vi "save_config.vi"() -> ()   [LabVIEW 2013]
uses:
  <vilib>/Analysis/Matrix/Datatypes/RealMatrix.ctl
  <vilib>/Analysis/Matrix/NI_Matrix.lvlib
panel:
  in  "Version":string="f"
  in  "Camera Serial":string="f"
  in  "Camera Model":string="f"
  in  "SOFT_VERSION":string="V2"
  in  "config Name":string="test2"
  in  "Config Directory":path=path "D:/CONFIGS_TIME_LAPSE"
  in  "USED_FILTERS":u8[](array[numeric])
  in  "USED_LEDS":bool[][](array[boolean])=[[FALSE, FALSE], [TRUE, TRUE]]
  in  "Nstart":u32=30 step=1
  in  "Non":u32=150 step=1
  in  "Noff":u32 step=1
  in  "BETWEEN_PAT":u32
  in  "NPAT":u32
  in  "BETWEEN_SCAN":u32
  in  "NSCAN":u32
  in  "XYPOS":T1=[[1.0, 1.0]]
  in  "STAGE_PORT":refnum<visa-resource-name>="COM1"
  in  "STAGE_SPEED":dbl
  in  "ROMODE":u32
  in  "BIN":u16
  in  "EXPT":dbl
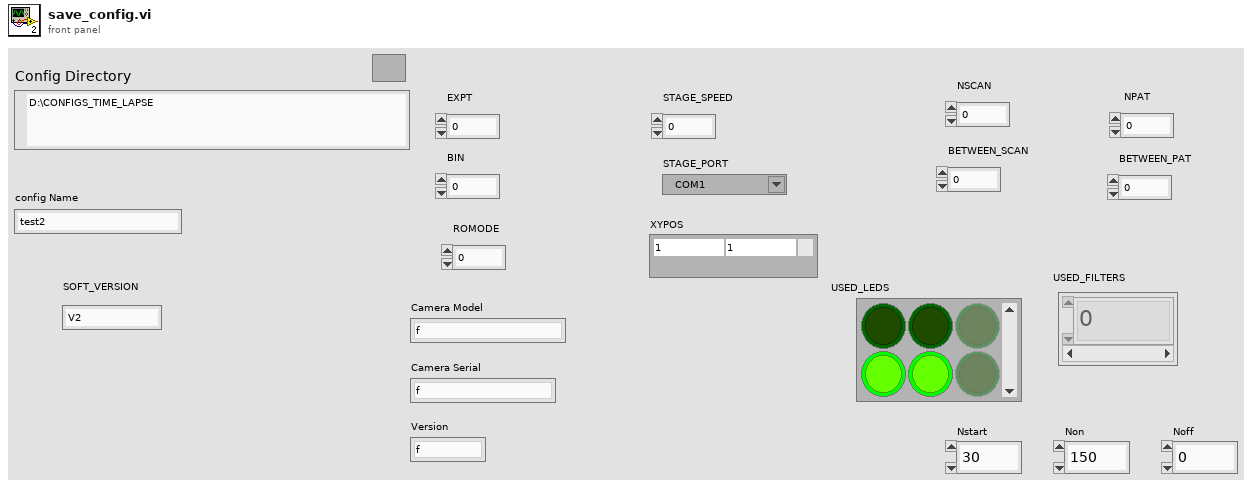
[diagram p1: front panel]
types:
  T1 = typedef "NI_Matrix.lvlib/RealMatrix.ctl" = dbl[][]
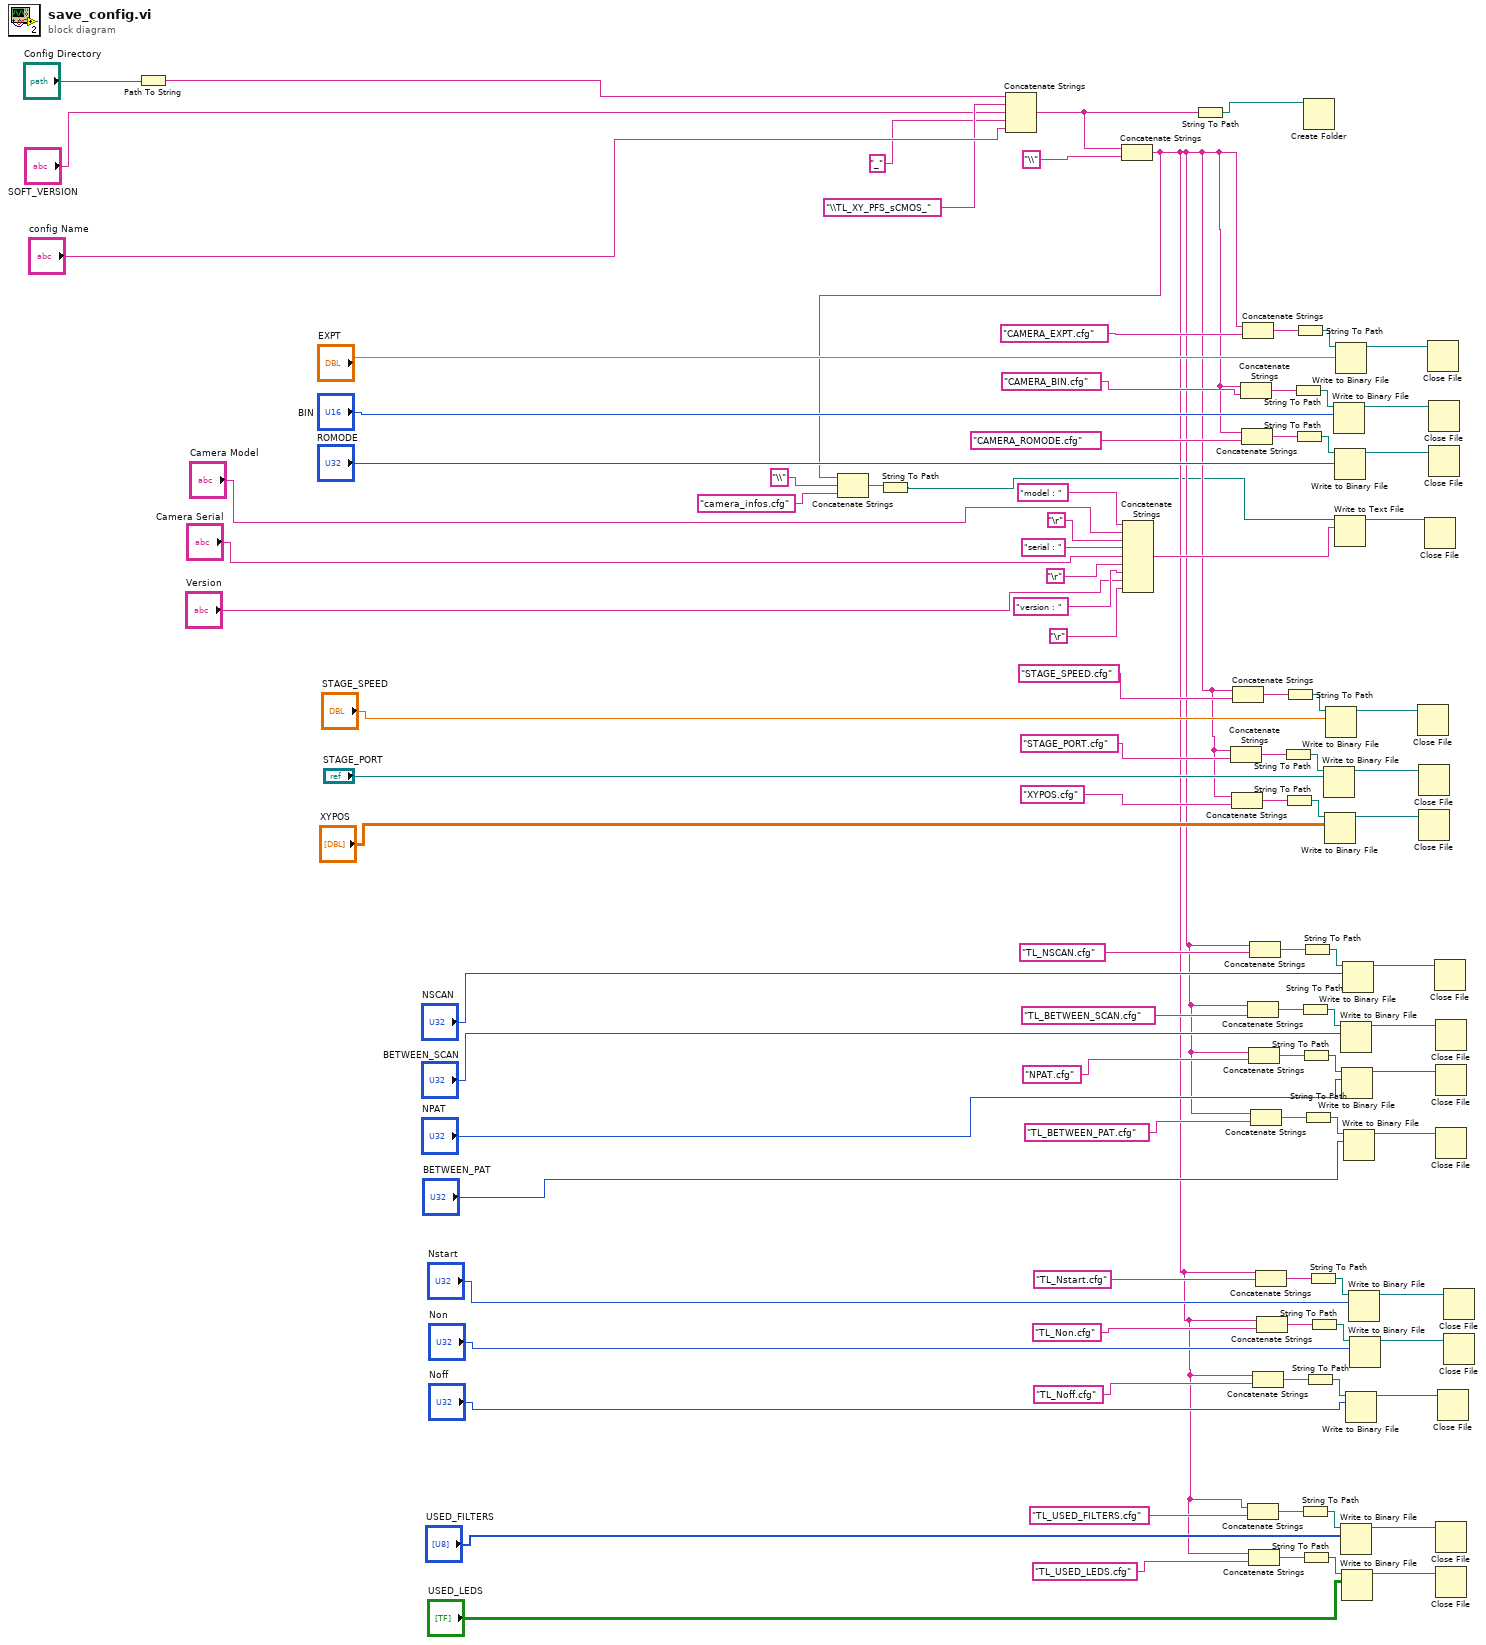
[diagram p0: block diagram]
diagram:
  n1 = Path To String(path="Config Directory") -> (string=w99:string)
  n2 = Concatenate Strings(w99, "\\TL_XY_PFS_sCMOS_", "SOFT_VERSION", "_", "config Name") -> (w92:string)
  n3 = Concatenate Strings(w92, "\\") -> (w5:string)
  n4 = Concatenate Strings(w5, "\\", "camera_infos.cfg") -> (w4:string)
  n5 = String To Path(string=w4) -> (path=w1:path)
  n6 = Concatenate Strings("model : ", "Camera Model", "\r", "serial : ", "Camera Serial", "\r", "version : ", "Version", "\r") -> (w70:string)
  n7 = String To Path(string=w92) -> (path=w98:path)
  n8 = Concatenate Strings(w5, "STAGE_PORT.cfg") -> (w64:string)
  n9 = Concatenate Strings(w5, "XYPOS.cfg") -> (w63:string)
  n10 = Concatenate Strings(w5, "STAGE_SPEED.cfg") -> (w65:string)
  n11 = Concatenate Strings(w5, "CAMERA_BIN.cfg") -> (w87:string)
  n12 = Concatenate Strings(w5, "CAMERA_ROMODE.cfg") -> (w82:string)
  n13 = Concatenate Strings(w5, "CAMERA_EXPT.cfg") -> (w88:string)
  n14 = Concatenate Strings(w5, "TL_BETWEEN_SCAN.cfg") -> (w49:string)
  n15 = Concatenate Strings(w5, "TL_USED_FILTERS.cfg") -> (w31:string)
  n16 = Concatenate Strings(w5, "NPAT.cfg") -> (w48:string)
  n17 = Concatenate Strings(w5, "TL_USED_LEDS.cfg") -> (w30:string)
  n18 = Concatenate Strings(w5, "TL_NSCAN.cfg") -> (w50:string)
  n19 = Concatenate Strings(w5, "TL_BETWEEN_PAT.cfg") -> (w41:string)
  n20 = Concatenate Strings(w5, "TL_Noff.cfg") -> (w32:string)
  n21 = Concatenate Strings(w5, "TL_Nstart.cfg") -> (w40:string)
  n22 = Concatenate Strings(w5, "TL_Non.cfg") -> (w39:string)
  n23 = String To Path(string=w64) -> (path=w61:path)
  n24 = String To Path(string=w63) -> (path=w60:path)
  n25 = String To Path(string=w65) -> (path=w62:path)
  n26 = String To Path(string=w87) -> (path=w86:path)
  n27 = String To Path(string=w82) -> (path=w81:path)
  n28 = String To Path(string=w88) -> (path=w90:path)
  n29 = String To Path(string=w49) -> (path=w46:path)
  n30 = String To Path(string=w31) -> (path=w28:path)
  n31 = String To Path(string=w48) -> (path=w45:path)
  n32 = String To Path(string=w30) -> (path=w27:path)
  n33 = String To Path(string=w50) -> (path=w47:path)
  n34 = String To Path(string=w41) -> (path=w38:path)
  n35 = Create Folder(path (use dialog)=w98) -> ()  [unwired: 2 in, 3 out]
  n36 = String To Path(string=w32) -> (path=w29:path)
  n37 = String To Path(string=w40) -> (path=w37:path)
  n38 = String To Path(string=w39) -> (path=w36:path)
  n39 = Write to Binary File(file (use dialog)=w61, data="STAGE_PORT") -> (refnum out=w58:refnum<file>)  [unwired: 4 in, 2 out]
  n40 = Write to Binary File(file (use dialog)=w60, data="XYPOS") -> (refnum out=w57:refnum<file>)  [unwired: 4 in, 2 out]
  n41 = Write to Binary File(file (use dialog)=w62, data="STAGE_SPEED") -> (refnum out=w59:refnum<file>)  [unwired: 4 in, 2 out]
  n42 = Write to Binary File(file (use dialog)=w86, data="BIN") -> (refnum out=w68:refnum<file>)  [unwired: 4 in, 2 out]
  n43 = Write to Binary File(file (use dialog)=w81, data="ROMODE") -> (refnum out=w67:refnum<file>)  [unwired: 4 in, 2 out]
  n44 = Write to Text File(file (use dialog)=w1, text=w70) -> (refnum out=w66:refnum<file>)  [unwired: 2 in, 2 out]
  n45 = Write to Binary File(file (use dialog)=w90, data="EXPT") -> (refnum out=w69:refnum<file>)  [unwired: 4 in, 2 out]
  n46 = Write to Binary File(file (use dialog)=w46, data="BETWEEN_SCAN") -> (refnum out=w43:refnum<file>)  [unwired: 4 in, 2 out]
  n47 = Write to Binary File(file (use dialog)=w28, data="USED_FILTERS") -> (refnum out=w25:refnum<file>)  [unwired: 4 in, 2 out]
  n48 = Write to Binary File(file (use dialog)=w45, data="NPAT") -> (refnum out=w42:refnum<file>)  [unwired: 4 in, 2 out]
  n49 = Write to Binary File(file (use dialog)=w27, data="USED_LEDS") -> (refnum out=w24:refnum<file>)  [unwired: 4 in, 2 out]
  n50 = Write to Binary File(file (use dialog)=w47, data="NSCAN") -> (refnum out=w44:refnum<file>)  [unwired: 4 in, 2 out]
  n51 = Write to Binary File(file (use dialog)=w38, data="BETWEEN_PAT") -> (refnum out=w35:refnum<file>)  [unwired: 4 in, 2 out]
  n52 = Write to Binary File(file (use dialog)=w29, data="Noff") -> (refnum out=w26:refnum<file>)  [unwired: 4 in, 2 out]
  n53 = Write to Binary File(file (use dialog)=w37, data="Nstart") -> (refnum out=w34:refnum<file>)  [unwired: 4 in, 2 out]
  n54 = Write to Binary File(file (use dialog)=w36, data="Non") -> (refnum out=w33:refnum<file>)  [unwired: 4 in, 2 out]
  n55 = Close File(refnum=w59) -> ()  [unwired: 1 in, 2 out]
  n56 = Close File(refnum=w58) -> ()  [unwired: 1 in, 2 out]
  n57 = Close File(refnum=w57) -> ()  [unwired: 1 in, 2 out]
  n58 = Close File(refnum=w66) -> ()  [unwired: 1 in, 2 out]
  n59 = Close File(refnum=w69) -> ()  [unwired: 1 in, 2 out]
  n60 = Close File(refnum=w68) -> ()  [unwired: 1 in, 2 out]
  n61 = Close File(refnum=w67) -> ()  [unwired: 1 in, 2 out]
  n62 = Close File(refnum=w44) -> ()  [unwired: 1 in, 2 out]
  n63 = Close File(refnum=w43) -> ()  [unwired: 1 in, 2 out]
  n64 = Close File(refnum=w42) -> ()  [unwired: 1 in, 2 out]
  n65 = Close File(refnum=w35) -> ()  [unwired: 1 in, 2 out]
  n66 = Close File(refnum=w25) -> ()  [unwired: 1 in, 2 out]
  n67 = Close File(refnum=w24) -> ()  [unwired: 1 in, 2 out]
  n68 = Close File(refnum=w26) -> ()  [unwired: 1 in, 2 out]
  n69 = Close File(refnum=w34) -> ()  [unwired: 1 in, 2 out]
  n70 = Close File(refnum=w33) -> ()  [unwired: 1 in, 2 out]
